vi "FATFS文件IO实验.vi"() -> ()   [LabVIEW 2011]
uses:
  <vilib>/STM32_DriverVI_Interface_F4/FATFS/Access (0;read-write)_F4.ctl
panel:
  out "文本":string
  in  "read":bool
  in  "write":bool
  out "大小（字节）":u32
  out "Status_Back":u16
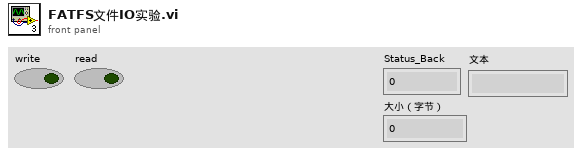
[diagram p1: front panel]
types:
  T1 = typedef "Access (0;read-write)_F4.ctl" = u8
  T2 = typedef "操作(0;open)_F4.ctl" = u8
  T3 = enum8{"P0", "P1", "P2", "P3", "P4", "P5", "P6", "P7", "P8", "P9", "P10", "P11", "P12", "P13", "P14", "P15"}
  T4 = enum8{"Port_A", "Port_B", "Port_C", "Port_D", "Port_E", "Port_F", "Port_G", "Port_H", "Port_I"}
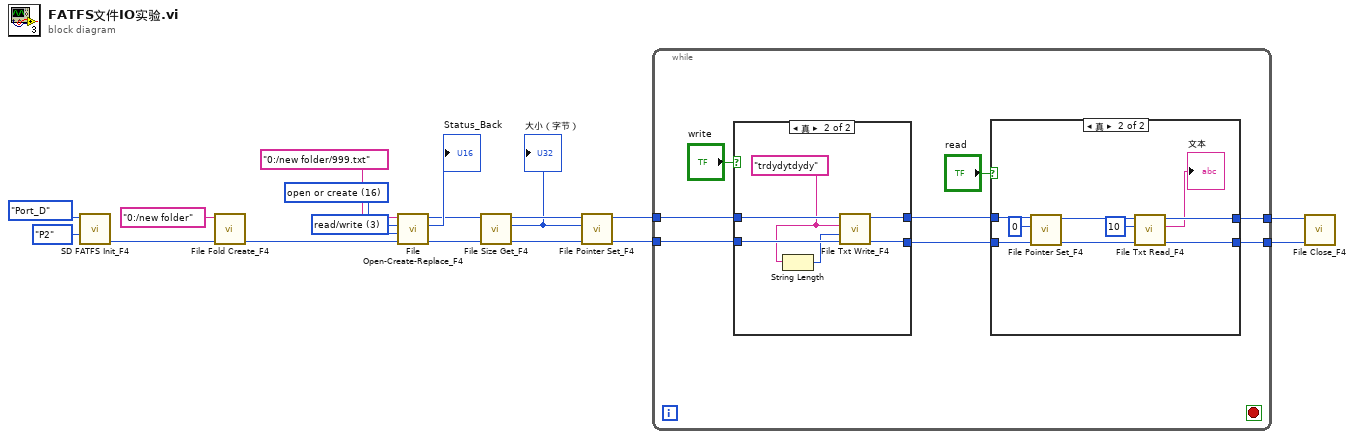
[diagram p0: block diagram]
diagram:
  w11 = T1 3 items=["read-only"=1, "write-only"=2, "read/write"=3] ("access (3:read/write)")
  w12 = T2 16 items=["open"=0, "create"=4, "open or create"=16, "replace or create"=8] ("Operate(3:open)")
  n1 = call <vilib>:"SD FATFS Init_F4.vi"("SD_CS_pin"=T3."P2", "SD_CS_PortX"=T4."Port_D") -> ("err_out"=w16:u8)  [unwired: 8 in, 1 out]
  n2 = call <vilib>:"File Fold Create_F4.vi"("err_in"=w16, "Fold Path"="0:/new folder") -> ("err_out"=w14:u8)  [unwired: 8 in, 1 out]
  n3 = call <vilib>:"File Open-Create-Replace_F4.vi"("err_in"=w14, "access (3:read/write)"=w11, "Operate(3:open)"=w12, "File Path"="0:/new folder/999.txt") -> ("err_out"=w9:u8, "Status_Back"=→"Status_Back":u16, "文件句柄输出"=w8:u16)  [unwired: 5 in]
  n4 = call <vilib>:"File Size Get_F4.vi"("err_in"=w9, "文件句柄输入"=w8) -> ("err_out"=w7:u8, "大小（字节）"=w5:u32, "文件句柄输出"=w6:u16)  [unwired: 7 in]
  "大小（字节）" <- w5
  n5 = call <vilib>:"File Pointer Set_F4.vi"("err_in"=w7, "偏移量（字节）"=w5, "文件句柄输入"=w6) -> ("err_out"=w4:u8, "文件句柄输出"=w3:u16)  [unwired: 6 in, 1 out]
  n6 = while {
    tunnel: w4 -> [w24]
    tunnel: w3 -> [w25]
    tunnel: [w20] -> w2
    tunnel: [w19] -> w1
    stop <- _ stop-if-true
    n7 = case shown="真" "write" {
      tunnel: w25 -> [_ w38]
      tunnel: w24 -> [_ w41]
      tunnel: [_ w40] -> w21
      tunnel: [_ w39] -> w22
      frame False {
      }
      frame True {
        w37 = "trdydytdydy" ("文本")
        n8 = String Length(string=w37) -> (length=w36:i32)
        n9 = call <vilib>:"File Txt Write_F4.vi"("err_in"=w41, "长度"=w36, "文本"=w37, "文件句柄输入"=w38) -> ("err_out"=w40:u8, "文件句柄输出"=w39:u16)  [unwired: 5 in, 1 out]
      }
    }
    n10 = case shown="真" "read" {
      tunnel: w22 -> [_ w34]
      tunnel: w21 -> [_ w35]
      tunnel: [_ w29] -> w20
      tunnel: [_ w28] -> w19
      frame False {
      }
      frame True {
        n11 = call <vilib>:"File Pointer Set_F4.vi"("err_in"=w35, "偏移量（字节）"=u32 0, "文件句柄输入"=w34) -> ("err_out"=w32:u8, "文件句柄输出"=w31:u16)  [unwired: 6 in, 1 out]
        n12 = call <vilib>:"File Txt Read_F4.vi"("err_in"=w32, "长度"=u16 10, "文件句柄输入"=w31) -> ("err_out"=w29:u8, "文本"=→"文本":string, "文件句柄输出"=w28:u16)  [unwired: 4 in, 2 out]
      }
    }
  }
  n13 = call <vilib>:"File Close_F4.vi"("err_in"=w2, "文件句柄输入"=w1) -> ()  [unwired: 8 in, 2 out]
